vi "Open Device.vi"(8 "error in (no error)":errorcluster, 9 "Serial Number":string, 10 "_Config File":path, 11 "Topas4 in":refnum<class "Topas4.lvclass">) -> (0 "error out":errorcluster, 3 "Topas4 out":refnum<class "Topas4.lvclass">)   [LabVIEW 2020, in "Topas4.lvclass"]
uses:
  Topas4.lvclass
  Topas4.lvclass/Topas4.ctl
  Topas4-LabVIEW-Driver/Library/Topas4.lvlib
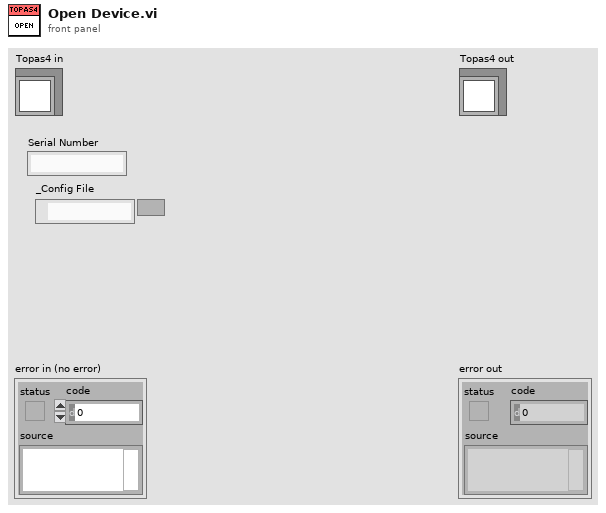
[diagram p1: front panel]
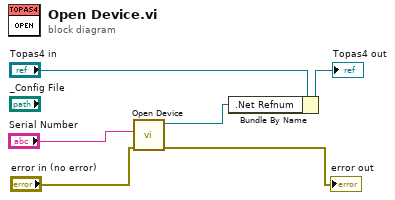
[diagram p0: block diagram]
diagram:
  n1 = call "Open Device.vi"("error in"="error in (no error)", "Serial Number"="Serial Number") -> ("error out"=→"error out":errorcluster, "reference out"=w1:refnum<k24>)  [unwired: 8 in]
  n2 = Bundle By Name(cluster="Topas4 in", ".Net Refnum"=w1) -> (→"Topas4 out":refnum<class "Topas4.lvclass">)
